vi "Joystick Rumble 2016.vi"   [LabVIEW 2015]
uses:
  Global Variables/Vision Processing Data.vi
  Global Variables/refnum names.vi
  <vilib>/Rock Robotics/WPI/Utilities/WPI_GetSetVariantRefNum.vi
  Global Variables/Settings.vi
  Global Variables/Calibrations.vi
  Global Variables/Temp Variables.vi
types:
  T1 = typedef "WPI_JoystickDevRef.ctl" = cluster{"Device":T2}
  T2 = typedef "WPI_JoystickDeviceEnum.ctl" = enum16{"USB 0", "USB 1", "USB 2", "USB 3", "USB 4", "USB 5"}
  T3 = cluster{"Distance (ft)":dbl, "Center":cluster{dbl, dbl}, "Normalized Rect":cluster{"Numeric":dbl, "Numeric 2":dbl, "Numeric 3":dbl, "Numeric 5":dbl}}[]
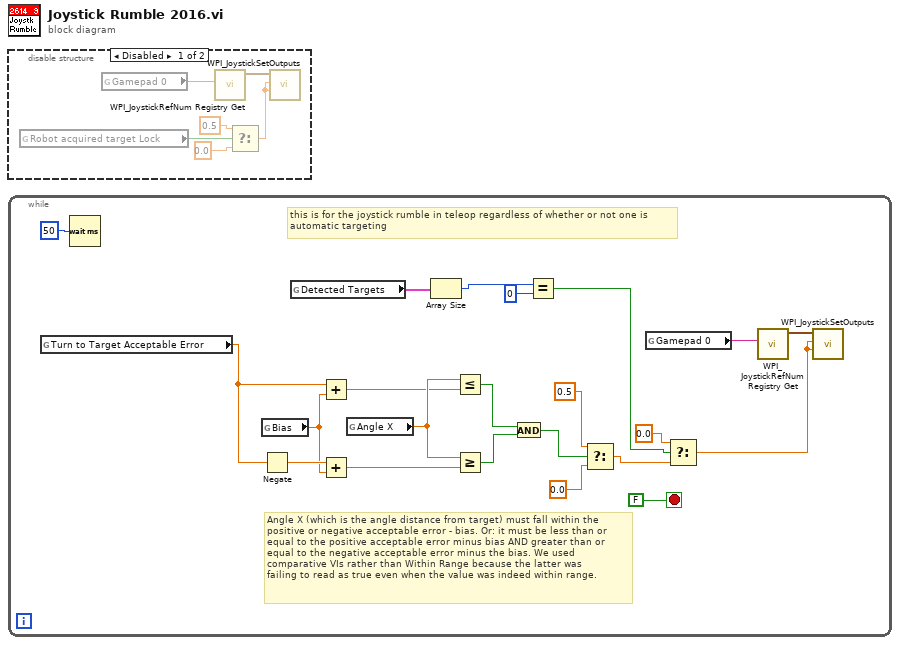
[diagram p0: block diagram]
diagram:
  n1 = disable-structure shown="Disabled" {
    frame Disabled {
      n2 = global read "Temp Variables.vi" "Robot acquired target Lock"() -> (w1:bool)
      n3 = global read "refnum names.vi" "Gamepad 0"() -> (w6:string)
      n4 = call <vilib>:"WPI_JoystickRefNum Registry Get.vi"("refnum name"=w6) -> ("JoystickDevRef"=w5:T1)  [unwired: 9 in, 1 out]
      n5 = Select(t=0.5, s=w1, f=0.0) -> (s? t:f=w2:dbl)
      n6 = call <vilib>:"WPI_JoystickSetOutputs.vi"("Right Rumble"=w2, "Left Rumble"=w2, "JoystickDevRef"=w5) -> ()  [unwired: 7 in, 2 out]
    }
    frame Enabled {
    }
  }
  n7 = while {
    stop <- FALSE stop-if-true
    # "Angle X (which is the angle distance from target) must fall within the\npositive or negative acceptable error - bias. Or: it must be less than or\nequal to the positive acceptable error minus bias AND greater than or\nequal to the negative acceptable error minus the bias. We used\ncomparative VIs rather than Within Range because the latter was\nfailing to read as true even when the value was indeed within range."
    # "this is for the joystick rumble in teleop regardless of whether or not one is\nautomatic targeting"
    n8 = global read "Settings.vi" "Turn to Target Acceptable Error"() -> (w18:dbl)
    n9 = Wait (ms)(milliseconds to wait=u32 50) -> ()  [unwired: 1 out]
    n10 = global read "Calibrations.vi" "Bias"() -> (w14:dbl)
    n11 = Negate(x=w18) -> (-x=w17:dbl)
    n12 = global read "Vision Processing Data.vi" "Detected Targets"() -> (w13:T3)
    n13 = Add(x=w18, y=w14) -> (x+y=w15:dbl)
    n14 = Add(x=w17, y=w14) -> (x+y=w16:dbl)
    n15 = global read "Vision Processing Data.vi" "Angle X"() -> (w19:dbl)
    n16 = Array Size(array=w13) -> (size(s)=w12:i32)
    n17 = Less Or Equal?(x=w19, y=w15) -> (x <= y?=w22:bool)
    n18 = Greater Or Equal?(x=w19, y=w16) -> (x >= y?=w21:bool)
    n19 = And(x=w22, y=w21) -> (x .and. y?=w20:bool)
    n20 = Equal?(x=w12, y=0) -> (x = y?=w9:bool)
    n21 = Select(t=0.5, s=w20, f=0.0) -> (s? t:f=w10:dbl)
    n22 = global read "refnum names.vi" "Gamepad 0"() -> (w28:string)
    n23 = Select(t=0.0, s=w9, f=w10) -> (s? t:f=w7:dbl)
    n24 = call <vilib>:"WPI_JoystickRefNum Registry Get.vi"("refnum name"=w28) -> ("JoystickDevRef"=w25:T1)  [unwired: 9 in, 1 out]
    n25 = call <vilib>:"WPI_JoystickSetOutputs.vi"("Right Rumble"=w7, "Left Rumble"=w7, "JoystickDevRef"=w25) -> ()  [unwired: 7 in, 2 out]
  }
